vi "Write read operation timeout.vi"(8 "error in (no error)":errorcluster, 10 "read operation timeout":i32, 11 "transmission data unit in":refnum<class "Transmission Data Unit.lvclass">) -> (0 "error out":errorcluster, 3 "transmission data unit out":refnum<class "Transmission Data Unit.lvclass">)   [LabVIEW 2021, in "Transmission Data Unit.lvclass"]
uses:
  Transmission Data Unit.lvclass
  Transmission Data Unit.lvclass/Transmission Data Unit.ctl
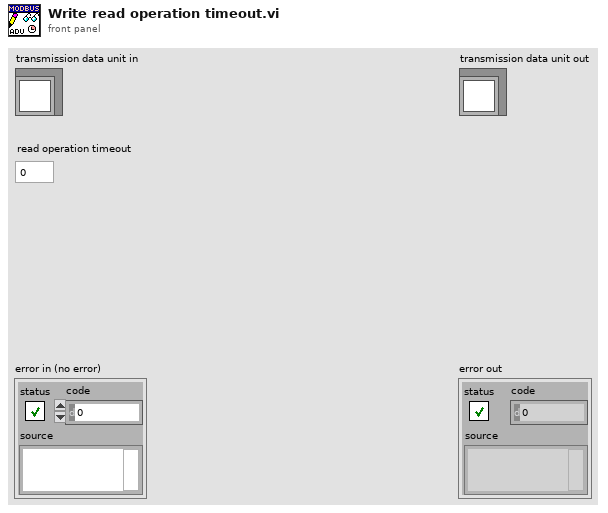
[diagram p1: front panel]
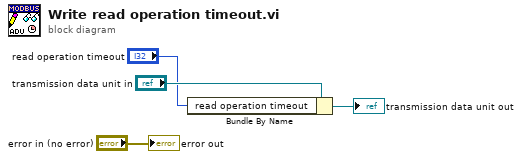
[diagram p0: block diagram]
diagram:
  n1 = Bundle By Name(cluster="transmission data unit in", "read operation timeout"="read operation timeout") -> (→"transmission data unit out":refnum<class "Transmission Data Unit.lvclass">)
  "error out" <- "error in (no error)"
